vi "PC_Offsets (DONE).vi"(7 "Saftey Factors":T1, 8 "Error In":errorcluster, 9 "Puck and Defender Inputs":T2, 10 "Table Walls Input":sgl[](array[numeric])) -> (0 "Error Out":errorcluster, 1 "Puck and Defender Output":T2, 2 "Table Walls Output":sgl[](array[numeric]))   [LabVIEW 2017]
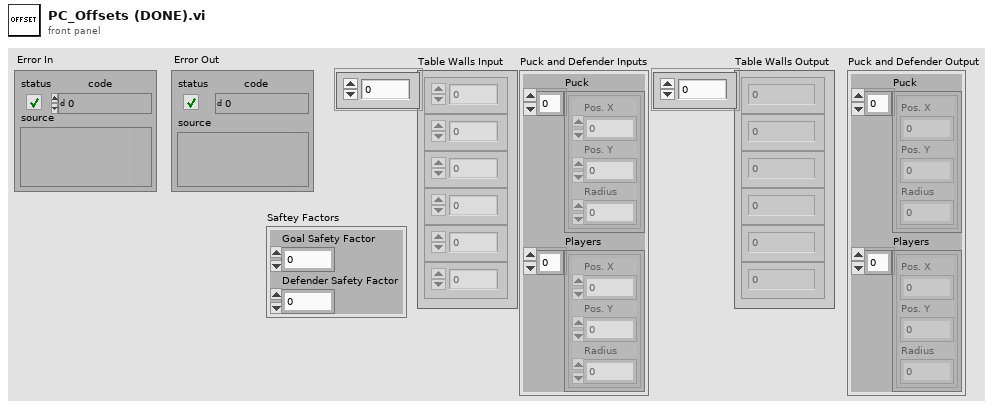
[diagram p1: front panel]
types:
  T1 = cluster{"Goal Safety Factor":dbl, "Defender Safety Factor":dbl}
  T2 = cluster{"Puck":cluster{"Pos. X":i32, "Pos. Y":i32, "Radius":i32}[], "Players":cluster{"Pos. X":i32, "Pos. Y":i32, "Radius":i32}[]}
  T3 = cluster{"Pos. X":i32, "Pos. Y":i32, "Radius":i32}[]
  T4 = cluster{"Pos. X":i32, "Pos. Y":i32, "Radius":i32}
  T5 = cluster{"Puck":cluster{"Pos. X":i32, "Pos. Y":i32, "Radius":i32}[], cluster{"Pos. X":i32, "Pos. Y":i32, "Radius":i32}[]}
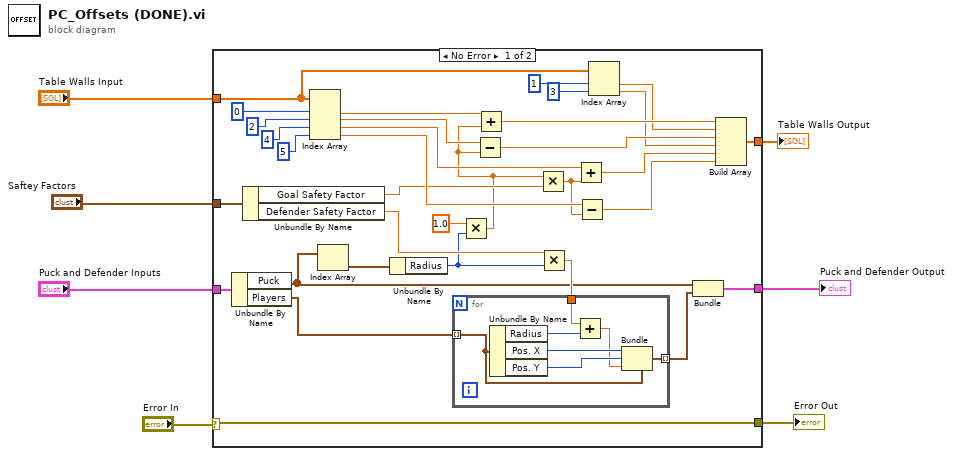
[diagram p0: block diagram]
diagram:
  n1 = case shown="No Error" "Error In" {
    selector: "Error In" -> [w14 w48]
    tunnel: "Puck and Defender Inputs" -> [w35 w49]
    tunnel: "Table Walls Input" -> [w27 w50]
    tunnel: [w19 w50] -> w5
    tunnel: [w15 w49] -> w4
    tunnel: [w14 w48] -> w2
    tunnel: "Saftey Factors" -> [w13 _]
    frame No Error {
      n2 = Unbundle By Name(w35) -> ("Puck"=w17:T3, "Players"=w18:T3)
      n3 = Unbundle By Name(w13) -> ("Goal Safety Factor"=w12:dbl, "Defender Safety Factor"=w11:dbl)
      n4 = Index Array(array=w27, index #1=0 ("index"), index #2=2 ("index"), index #3=4 ("index"), index #4=5 ("index")) -> (element #1=w34:sgl, element #2=w33:sgl, element #3=w32:sgl, element #4=w31:sgl)
      n5 = Index Array(array=w17) -> (element=w36:T4)  [unwired: 1 in]
      n6 = Unbundle By Name(w36) -> ("Radius"=w10:i32)
      n7 = Multiply(x=1.0, y=w10) -> (x*y=w9:dbl)
      n8 = Subtract(x=w33, y=w9) -> (x-y=w23:dbl)
      n9 = Add(x=w34, y=w9) -> (x+y=w28:dbl)
      n10 = Multiply(x=w9, y=w12) -> (x*y=w30:dbl)
      n11 = Multiply(x=w11, y=w10) -> (x*y=w29:dbl)
      n12 = for {
        tunnel: w18 -> [w41] mode=indexing
        tunnel: w29 -> [w46]
        tunnel: [w42] -> w16 mode=indexing
        n13 = Unbundle By Name(w41) -> ("Radius"=w47:i32, "Pos. X"=w45:i32, "Pos. Y"=w44:i32)
        n14 = Add(x=w46, y=w47) -> (x+y=w43:dbl)
        n15 = Bundle(cluster=w41, "Pos. X"=w45, "Pos. Y"=w44, "Radius"=w43) -> (w42:T4)
      }
      n16 = Add(x=w32, y=w30) -> (x+y=w21:dbl)
      n17 = Subtract(x=w31, y=w30) -> (x-y=w20:dbl)
      n18 = Index Array(array=w27, index #1=1 ("index"), index #2=3 ("index")) -> (element #1=w24:sgl, element #2=w22:sgl)
      n19 = Bundle("Puck"=w17, w16) -> (w15:T5)  [unwired: 1 in]
      n20 = Build Array(w28, w24, w23, w22, w21, w20) -> (w19:dbl[])
    }
    frame Error {
    }
  }
  "Error Out" <- w2
  "Table Walls Output" <- w5
  "Puck and Defender Output" <- w4
